vi "Extract RT File Data.vi"(7 "Data Cluster In":T1, 8 "Error In":errorcluster, 9 "Cancellled?":bool, 10 "Exists?":bool, 11 "Folder Path":path) -> (0 "Error Out":errorcluster, 5 "Data Cluster Out":T1)   [LabVIEW 2021, in "Test Configuration.lvlib"]
doc: "<b>Note:</b> This VI was modified by the <b>Validate DQMH Module</b> tool to turn off automatic error handling."
uses:
  Test Configuration.lvlib
  Module Data--cluster.ctl
  Configuration/All Interface Data.ctl
  Configuration/DO Channel's.ctl
  Configuration/Analog Input Single Channel Data--Cluster.ctl
  Configuration/Config-Channel Type.ctl
  Configuration/Channel Sub-Type.ctl
  Analog Output/Controls/AO Timing Cluster.ctl
  Host-Control's/Module ID Action Enum.ctl
  Host-Control's/HW Name Enum.ctl
  <vilib>/Utility/xml.llb/Read From XML File.vi
  <vilib>/Utility/xml.llb/Read From XML File(string).vi
  <vilib>/addons/_JKI.lib/Serialization/JSON/Library/Flatten To JSON String.vi
  Configuration/Configuration.lvlib
panel:
  out "filename without extension":string
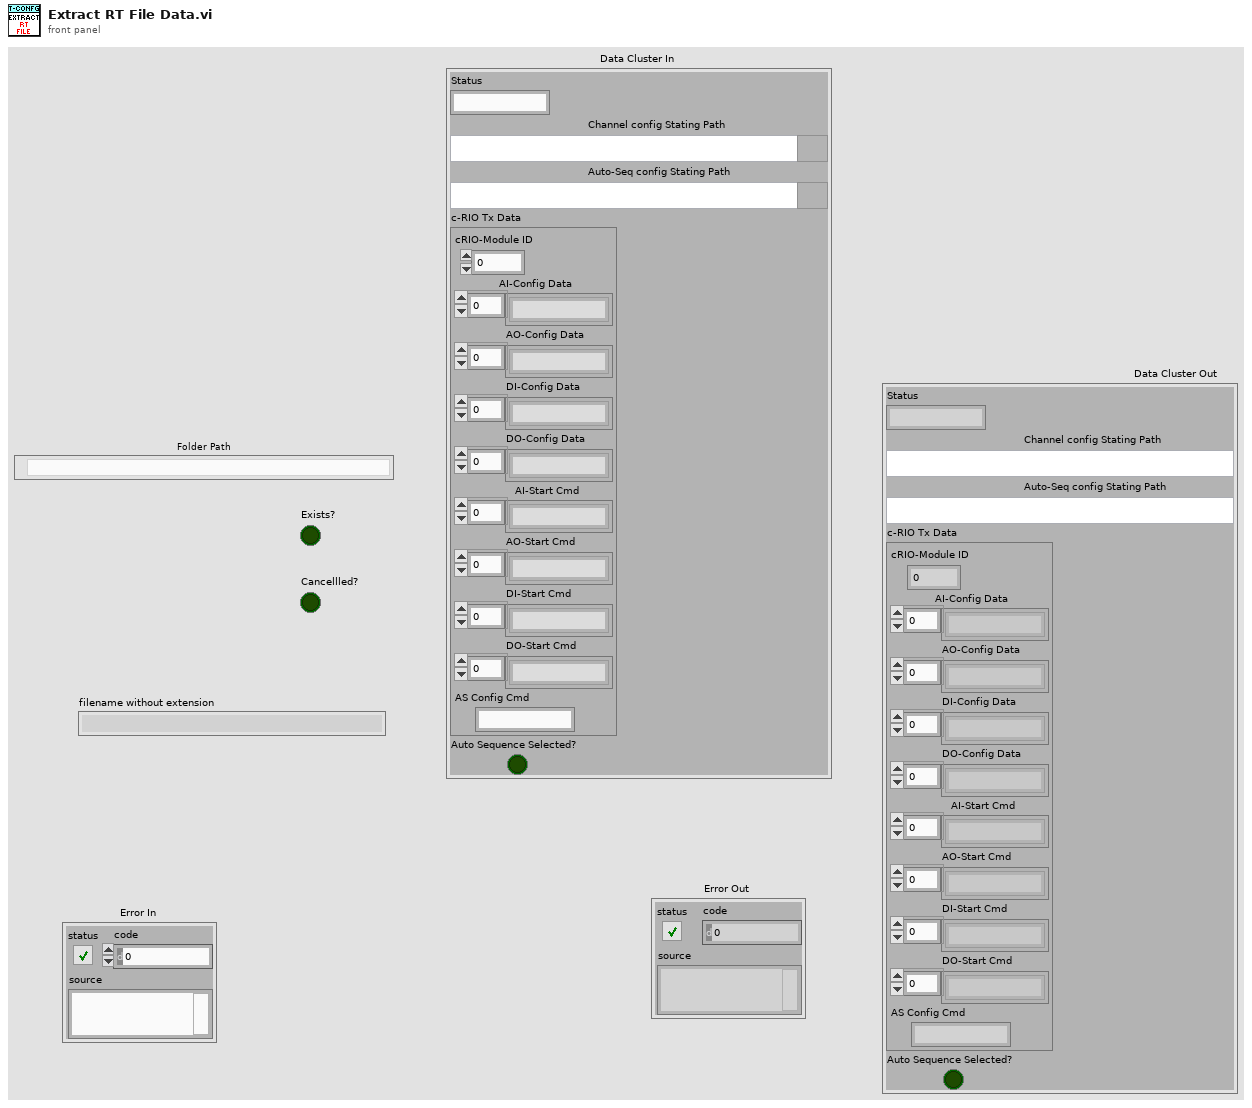
[diagram p1: front panel]
types:
  T1 = typedef "Test Configuration.lvlib/Module Data--cluster.ctl" = cluster{"Status":string, "Channel config Stating Path":path, "Auto-Seq config Stating Path":path, "c-RIO Tx Data":cluster{"cRIO-Module ID":i32, "AI-Config Data":string[], "AO-Config Data":string[], "DI-Config Data":string[], "DO-Config Data":string[], "AI-Start Cmd":string[], "AO-Start Cmd":string[], "DI-Start Cmd":string[], "DO-Start Cmd":string[], "AS Config Cmd":string}, "Auto Sequence Selected?":bool}
  T2 = typedef "Configuration.lvlib/All Interface Data.ctl" = cluster{"DI Config Data":T3, "DO Config Data":T3, "AI Config Data's":cluster{"Module Name":string, "AI Channel's Data":T4[], "Analog Input Timing":T7}[]}
  T3 = typedef "Configuration.lvlib/DO Channel's.ctl" = cluster{"Channel Name":string, "Identification Name":string, "Data":u8[], "Enabled?":bool}[]
  T4 = typedef "Configuration.lvlib/Analog Input Single Channel Data--Cluster.ctl" = cluster{"Channel Name":string, "Identification Name":string, "Channel Type":T5, "Sub-Type":T6, "Data":string, "Enabled?":bool}
  T5 = typedef "Configuration.lvlib/Config-Channel Type.ctl" = enum16{"Voltage", "Current", "Thermocouple", "Acclerometer"}
  T6 = typedef "Configuration.lvlib/Channel Sub-Type.ctl" = enum16{"None", "Pressure", "Force"}
  T7 = typedef "AO Timing Cluster.ctl" = cluster{"samples per channel":i32, "sample mode":i32, "Sampling Rate":dbl}
  T8 = typedef "HW Name Enum.ctl" = enum16{"Capsule-1", "Capsule-2", "Capsule-3", "Capsule-4", "sb-RIO", "Safety", "Release"}
  T9 = typedef "Module ID Action Enum.ctl" = enum16{"Init", "Insert", "Get a ID", "Get all ID"}
  T10 = cluster{"Module Name":string, "AI Channel's Data":T4[], "Analog Input Timing":T7}[]
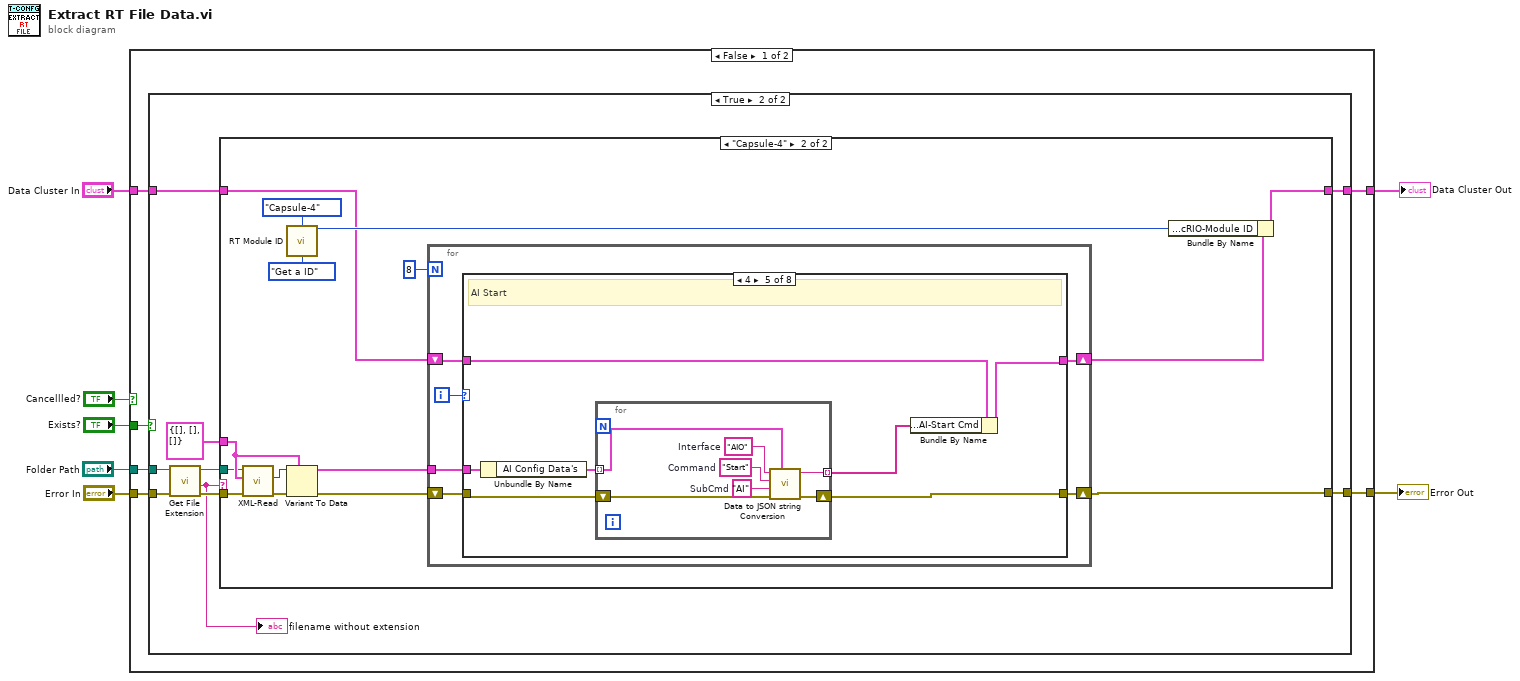
[diagram p0: block diagram]
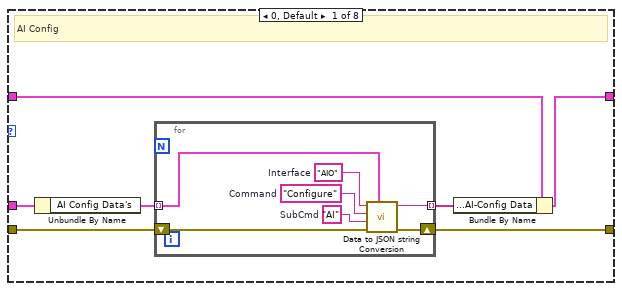
[diagram p4: hidden frame]
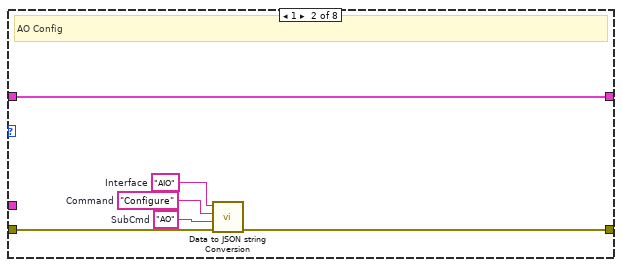
[diagram p5: hidden frame]
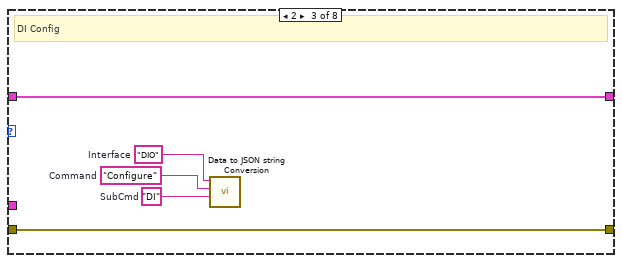
[diagram p6: hidden frame]
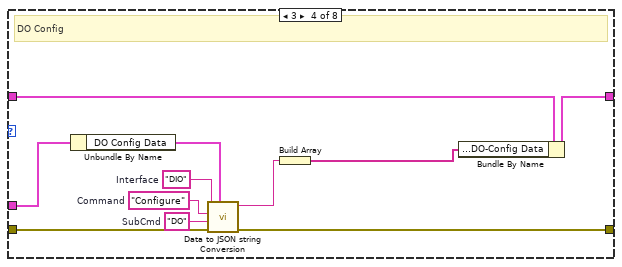
[diagram p7: hidden frame]
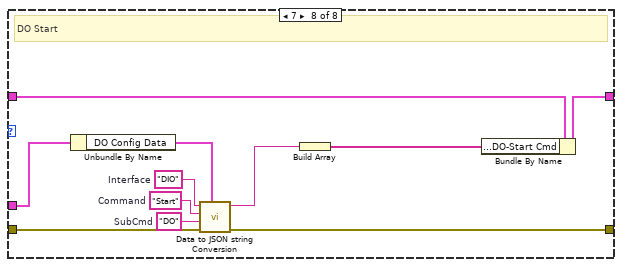
[diagram p10: hidden frame]
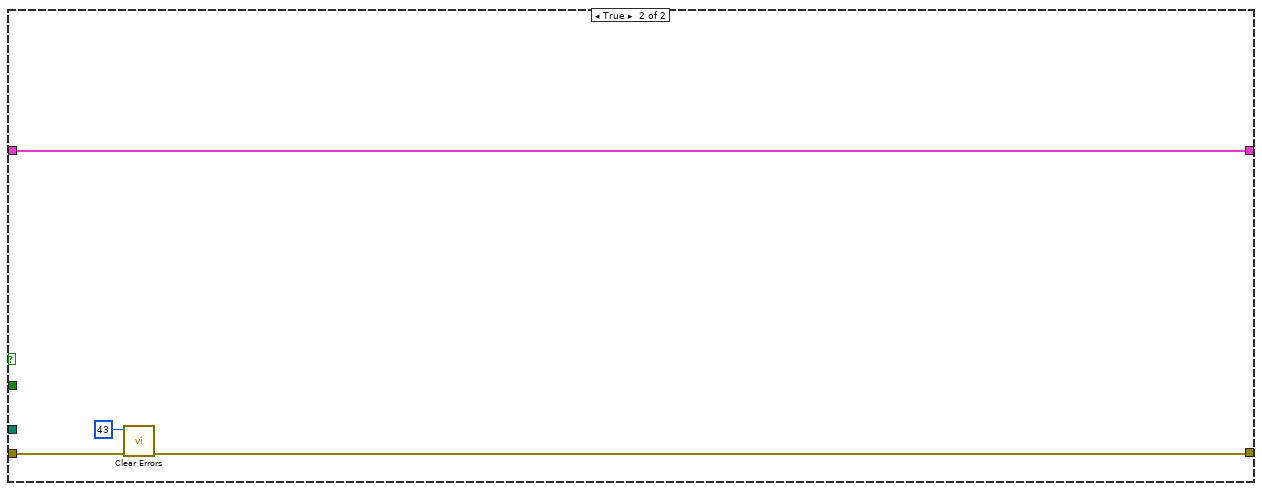
[diagram p11: hidden frame]
diagram:
  n1 = case shown="False" "Cancellled?" {
    tunnel: "Error In" -> [w13 w114]
    tunnel: [w12 w113] -> w3
    tunnel: "Folder Path" -> [w10 _]
    tunnel: "Exists?" -> [w11 _]
    tunnel: "Data Cluster In" -> [w9 w116]
    tunnel: [w8 w116] -> w1
    frame False {
      n2 = case shown="True" w11 {
        tunnel: w13 -> [w15 w19]
        tunnel: [w15 w24] -> w12
        tunnel: w10 -> [_ w20]
        tunnel: w9 -> [w14 w17]
        tunnel: [w14 w16] -> w8
        frame False {
        }
        frame True {
          n3 = call <vilib>:"Get File Extension.vi"("error in (no error)"=w19, "file"=w20) -> ("error out"=w21:errorcluster, "filename without extension"=w18:string, "dup file"=w22:path)  [unwired: 5 in, 2 out]
          "filename without extension" <- w18
          n4 = case shown="\"Capsule-4\"" w18 {
            tunnel: [w26 w33] -> w24
            tunnel: w21 -> [w26 w29]
            tunnel: w22 -> [_ w30]
            tunnel: T2 {"DI Config Data"=[], "DO Config Data"=[], "AI Config Data's"=[]} ("Interface Data") -> [_ w31]
            tunnel: w17 -> [w25 w37]
            tunnel: [w25 w38] -> w16
            frame Default {
            }
            frame "Capsule-4" {
              n5 = call "XML-Read.vi"("error in (no error)"=w29, "Data"=w31, "XML File Path"=w30) -> ("error out"=w27:errorcluster, "Data Out"=w28:variant)  [unwired: 6 in, 1 out]
              n6 = call "RT Module ID.vi"("HW Name"=HW_Name_Enum."Capsule-4", "Action"=Module_ID_Action_Enum."Get a ID") -> ("Module Id Out"=w39:i32)  [unwired: 10 in, 3 out]
              n7 = Variant To Data(error in=w27, type=w31, Variant=w28) -> (data=w36:T2, error out=w34:errorcluster)
              n8 = for {
                N: 8 -> [_]
                tunnel: w36 -> [w46]
                shift-right: [w43] -> w32
                shift-left: w37 -> [w42]
                shift-right: [w44] -> w33
                shift-left: w34 -> [w45]
                i -> [w47]
                n9 = case shown="4" w47 {
                  tunnel: w46 -> [w54 _ _ w78 w84 _ _ w104]
                  tunnel: w45 -> [w53 w64 w71 w80 w88 w98 w100 w108]
                  tunnel: [w52 w63 w71 w79 w87 w98 w100 w107] -> w44
                  tunnel: [w50 w62 w72 w75 w85 w99 w101 w105] -> w43
                  tunnel: w42 -> [w51 w62 w72 w76 w86 w99 w101 w106]
                  frame 0, Default {
                    # "AI Config"
                    n10 = Unbundle By Name(w54) -> ("AI Config Data's"=w48:T10)
                    n11 = for {
                      tunnel: [w56] -> w49 mode=indexing
                      tunnel: w48 -> [w55] mode=indexing
                      shift-right: [w57] -> w52
                      shift-left: w53 -> [w58]
                      w61 = "AI"  # SubCmd
                      w60 = "Configure"  # Command
                      w59 = "AIO"  # Interface
                      n12 = call "Data to JSON string Conversion.vi"("Data"=w55, "error in"=w58, "SubCmd"=w61, "Command"=w60, "Interface"=w59) -> ("error out"=w57:errorcluster, "Cmd String"=w56:string)  [unwired: 5 in]
                    }
                    n13 = Bundle By Name(cluster=w51, "c-RIO Tx Data.AI-Config Data"=w49) -> (w50:T1)
                  }
                  frame 1 {
                    w67 = "AO"  # SubCmd
                    w66 = "Configure"  # Command
                    w65 = "AIO"  # Interface
                    # "AO Config"
                    n14 = call "Data to JSON string Conversion.vi"("error in"=w64, "SubCmd"=w67, "Command"=w66, "Interface"=w65) -> ("error out"=w63:errorcluster)  [unwired: 6 in, 1 out]
                  }
                  frame 2 {
                    w70 = "DI"  # SubCmd
                    w69 = "Configure"  # Command
                    w68 = "DIO"  # Interface
                    # "DI Config"
                    n15 = call "Data to JSON string Conversion.vi"("SubCmd"=w70, "Command"=w69, "Interface"=w68) -> ()  [unwired: 7 in, 2 out]
                  }
                  frame 3 {
                    w83 = "DO"  # SubCmd
                    w82 = "Configure"  # Command
                    w81 = "DIO"  # Interface
                    # "DO Config"
                    n16 = Unbundle By Name(w78) -> ("DO Config Data"=w77:T3)
                    n17 = call "Data to JSON string Conversion.vi"("Data"=w77, "error in"=w80, "SubCmd"=w83, "Command"=w82, "Interface"=w81) -> ("error out"=w79:errorcluster, "Cmd String"=w74:string)  [unwired: 5 in]
                    n18 = Build Array(w74) -> (w73:string[])
                    n19 = Bundle By Name(cluster=w76, "c-RIO Tx Data.DO-Config Data"=w73) -> (w75:T1)
                  }
                  frame 4 {
                    # "AI Start"
                    n20 = Unbundle By Name(w84) -> ("AI Config Data's"=w90:T10)
                    n21 = for {
                      tunnel: w90 -> [w91] mode=indexing
                      tunnel: [w94] -> w89 mode=indexing
                      shift-right: [w92] -> w87
                      shift-left: w88 -> [w93]
                      w97 = "AI"  # SubCmd
                      w96 = "Start"  # Command
                      w95 = "AIO"  # Interface
                      n22 = call "Data to JSON string Conversion.vi"("Data"=w91, "error in"=w93, "SubCmd"=w97, "Command"=w96, "Interface"=w95) -> ("error out"=w92:errorcluster, "Cmd String"=w94:string)  [unwired: 5 in]
                    }
                    n23 = Bundle By Name(cluster=w86, "c-RIO Tx Data.AI-Start Cmd"=w89) -> (w85:T1)
                  }
                  frame 5 {
                    # "AO Start"
                  }
                  frame 6 {
                    # "DI Start"
                  }
                  frame 7 {
                    w112 = "DO"  # SubCmd
                    w111 = "Start"  # Command
                    w110 = "DIO"  # Interface
                    # "DO Start"
                    n24 = Unbundle By Name(w104) -> ("DO Config Data"=w109:T3)
                    n25 = call "Data to JSON string Conversion.vi"("Data"=w109, "error in"=w108, "SubCmd"=w112, "Command"=w111, "Interface"=w110) -> ("error out"=w107:errorcluster, "Cmd String"=w103:string)  [unwired: 5 in]
                    n26 = Build Array(w103) -> (w102:string[])
                    n27 = Bundle By Name(cluster=w106, "c-RIO Tx Data.DO-Start Cmd"=w102) -> (w105:T1)
                  }
                }
              }
              n28 = Bundle By Name(cluster=w32, "c-RIO Tx Data.cRIO-Module ID"=w39) -> (w38:T1)
            }
          }
        }
      }
    }
    frame True {
      n29 = call <vilib>:"Clear Errors.vi"("error in (no error)"=w114, "specific error code to clear (0: all)"=43) -> ("error out"=w113:errorcluster)  [unwired: 4 in, 1 out]
    }
  }
  "Error Out" <- w3
  "Data Cluster Out" <- w1
